vi "Set Scale.vi"(6 "Sensor ID (For Sensor Type)":string, 8 "error in (no error)":errorcluster, 9 "Params (Not Sensor)":dbl[](array[numeric]), 10 "Scale Type":T1, 11 "Channel in":refnum<class "Channel.lvclass">) -> (0 "error out":errorcluster, 3 "Channel out":refnum<class "Channel.lvclass">)   [LabVIEW 2020, in "VolatusConfig.lvlib" / "Channel.lvclass"]
uses:
  Channel.lvclass
  Channel.lvclass/Channel.ctl
  Scale/Scale.lvclass
  VolatusConfigElement/VolatusConfigElement.lvclass
  C:/dev/lv20CE/relink/lv-volatus/VolatusConfig/VolatusConfigElement/VolatusConfigElement.lvclass
  Scale Type.ctl
  VolatusConfig.lvlib
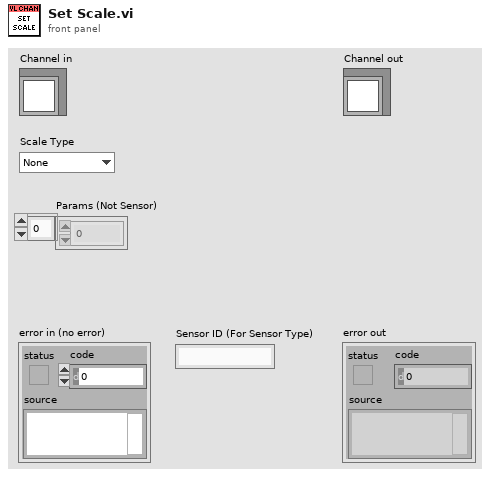
[diagram p1: front panel]
types:
  T1 = typedef "VolatusConfig.lvlib/Scale Type.ctl" = enum16{"None", "Sensor", "Polynomial", "Threshold", "Invert Bool"}
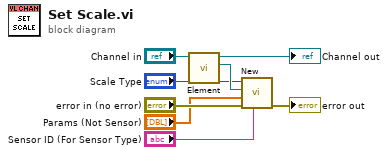
[diagram p0: block diagram]
diagram:
  n1 = call "Element.vi"("VolatusConfigElement in"="Channel in") -> ("Element"=w6:refnum<class "Config Element.lvclass">, "VolatusConfigElement out"=→"Channel out":refnum<class "Channel.lvclass">)  [unwired: 9 in]
  n2 = call "New.vi"("Sensor ID (For Sensor Type)"="Sensor ID (For Sensor Type)", "error in (no error)"="error in (no error)", "Scale Params (Not Sensor)"="Params (Not Sensor)", "Parent"=w6, "Scale Type"="Scale Type") -> ("error out"=→"error out":errorcluster)  [unwired: 5 in, 1 out]
